vi "routes_n_m-optimised with LUT.vi"(6 "LUT in":T1[](array[typedef]), 8 "error in (no error)":errorcluster, 9 "recursivity counter in":u32, 10 "m = number of nodes (horizontal)":u64, 11 "n = number of nodes (vertical)":u64) -> (0 "error out":errorcluster, 1 "recursivity counter out":u32, 2 "no. of LUT elements":i32, 3 "r(n,m)= number of routes":u64, 4 "LUT out":T1[](array[typedef]))   [LabVIEW 2021, in "Project Euler.lvlib"]
uses:
  Project Euler.lvlib
  LUT_element.ctl
panel:
  # "Development\ncontrols/indicators useful for development and testing, but which are not outputs of the VI"
  # "Input\nInputs to the VI"
  # "Output\nOutputs of the VI"
  # "Description\n\nBlank VI with error handling case. \n\nSummarize the use of this VI in this space."
  # "r(15,15) = 40,116,600\nr(16,16) = 155,117,520\nr(17,17) = 601,080,390"
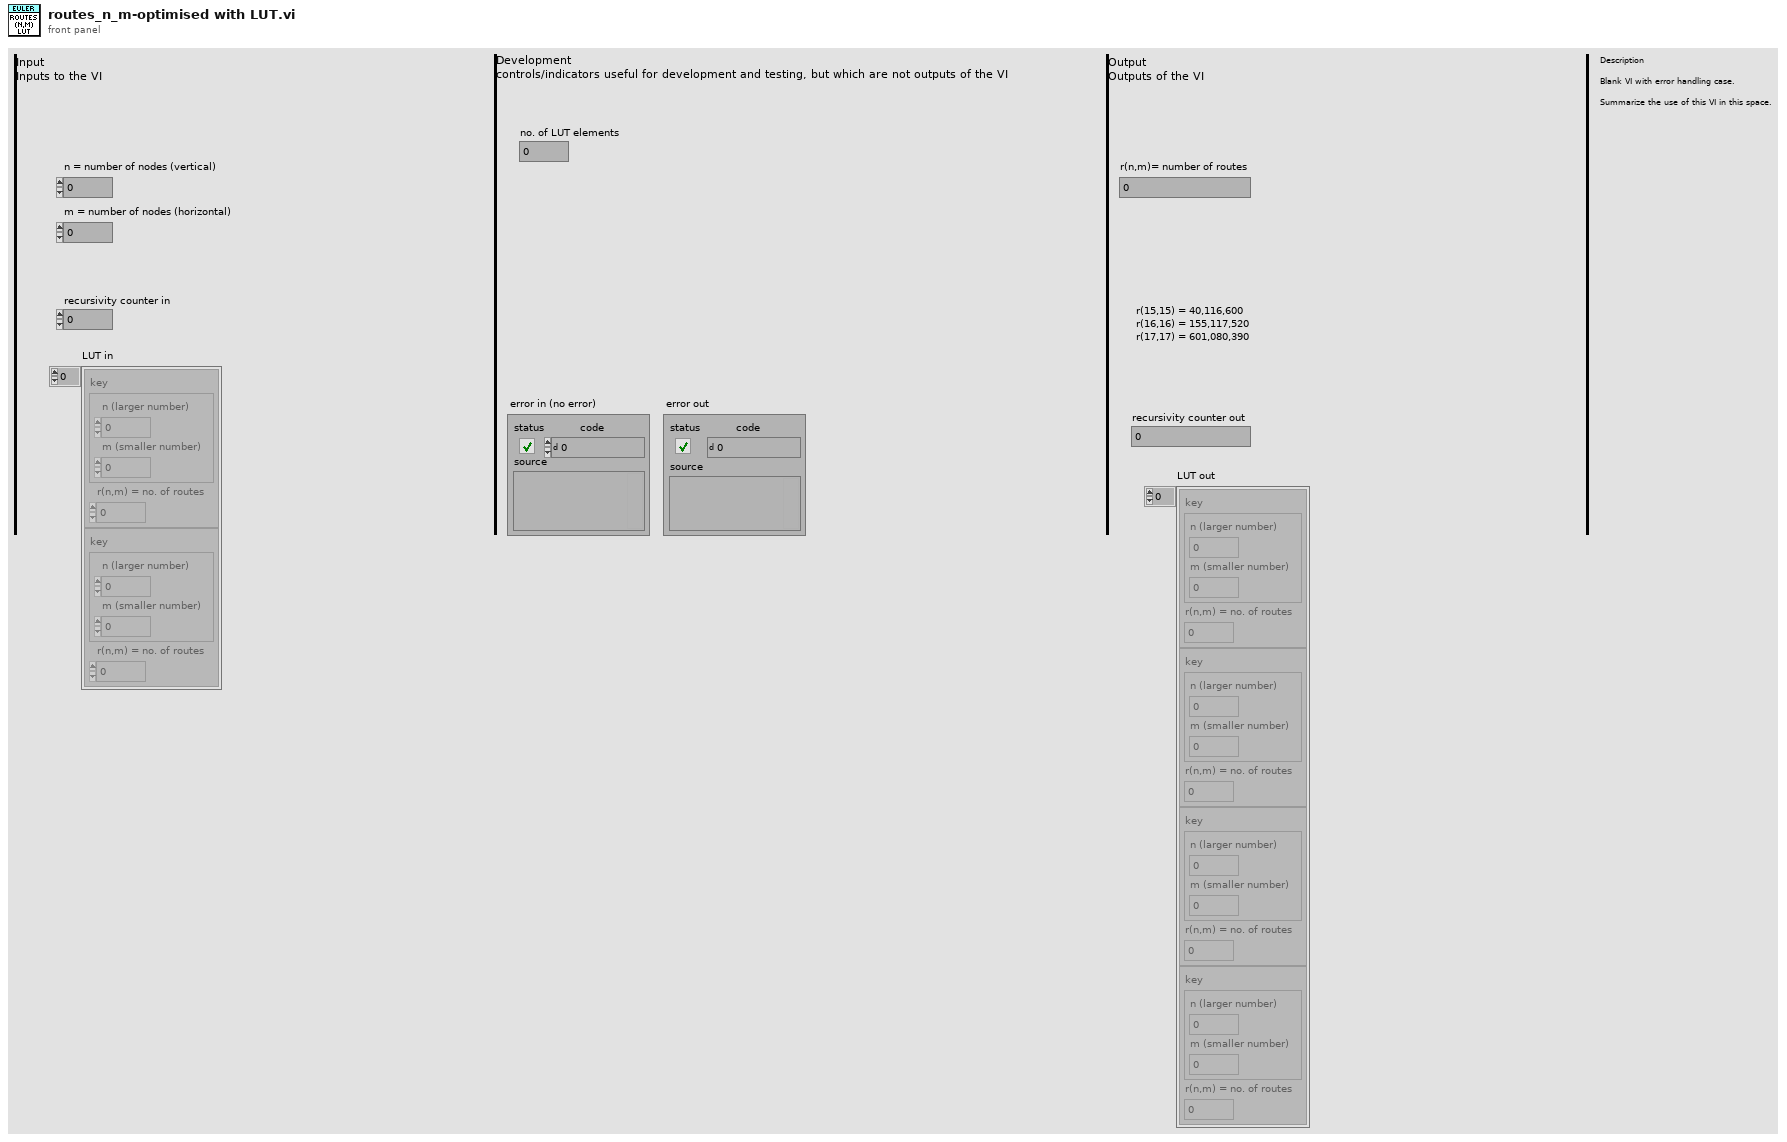
[diagram p1: front panel]
types:
  T1 = typedef "Project Euler.lvlib/LUT_element.ctl" = cluster{"key":cluster{"n (larger number)":u64, "m (smaller number)":u64}, "r(n,m) = no. of routes":u64}
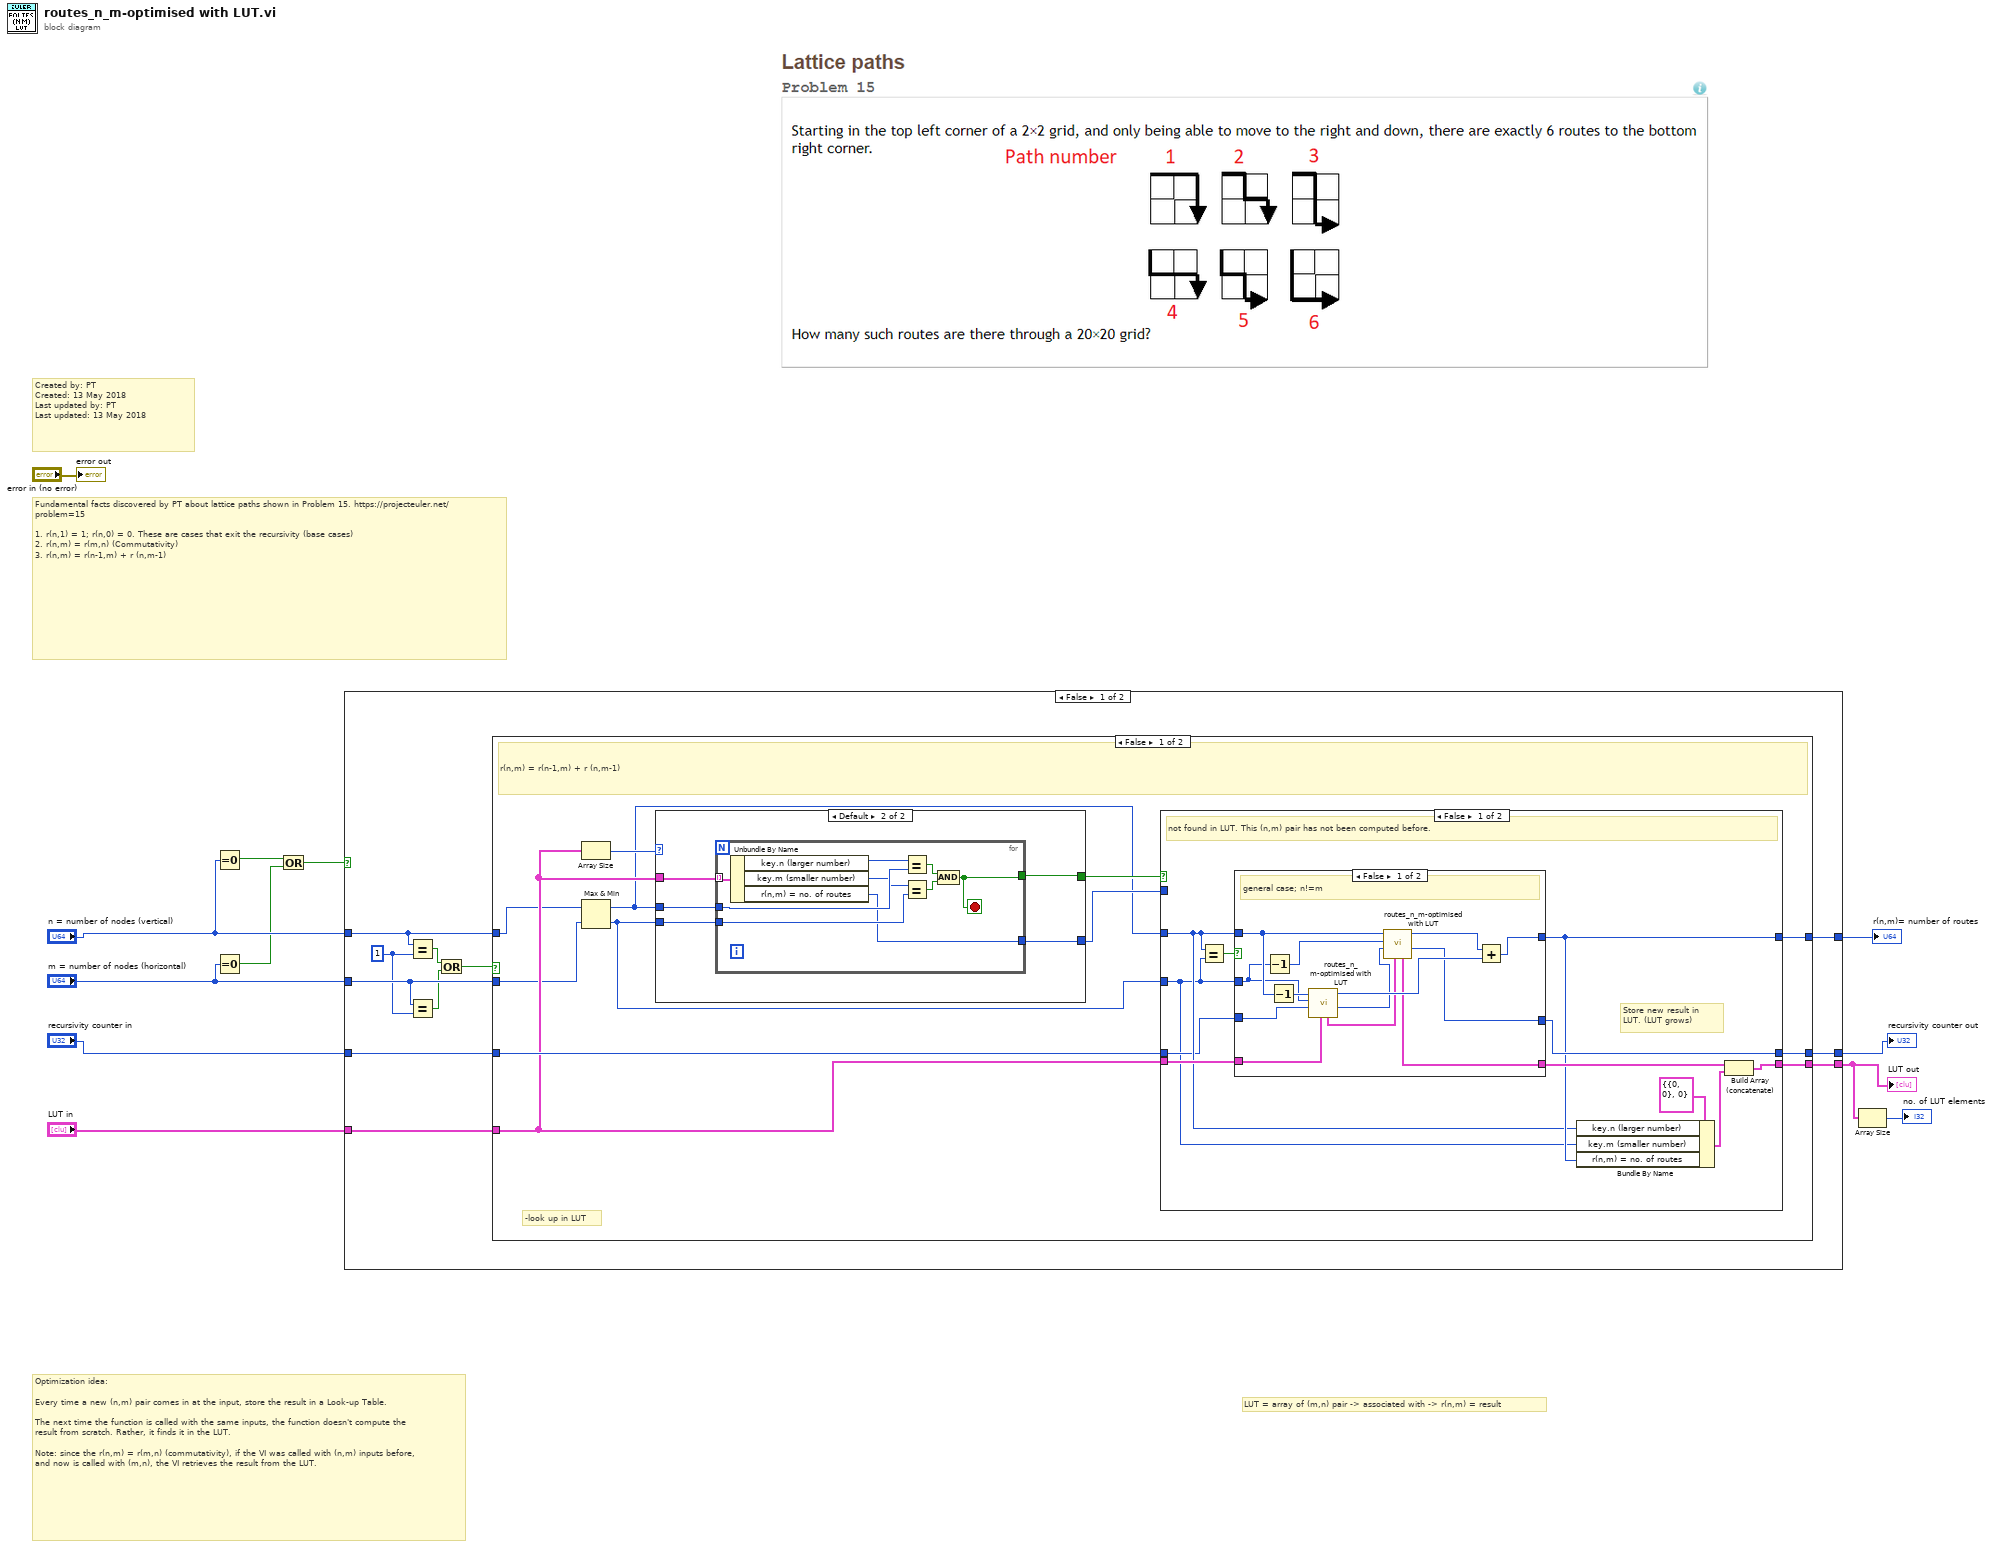
[diagram p0: block diagram]
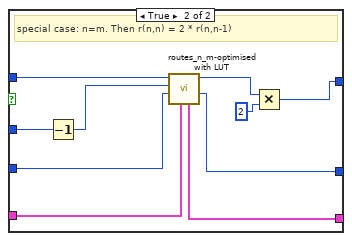
[diagram p3: hidden frame]
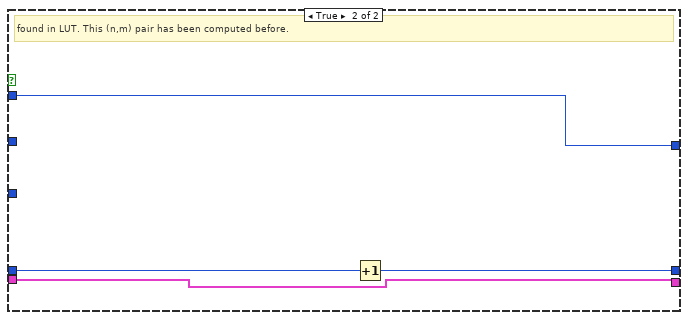
[diagram p4: hidden frame]
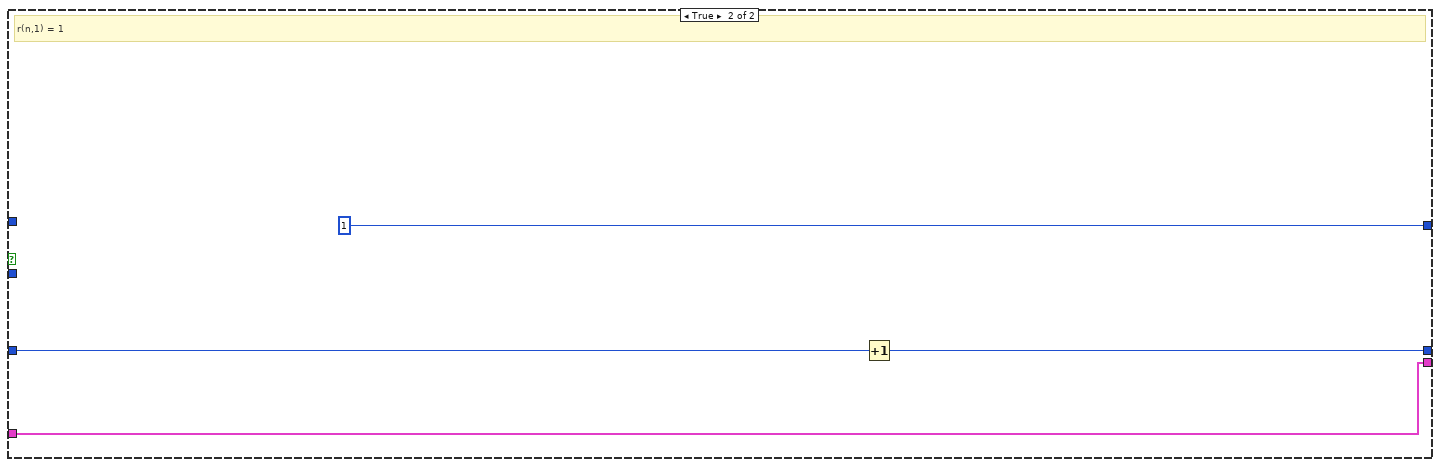
[diagram p5: hidden frame]
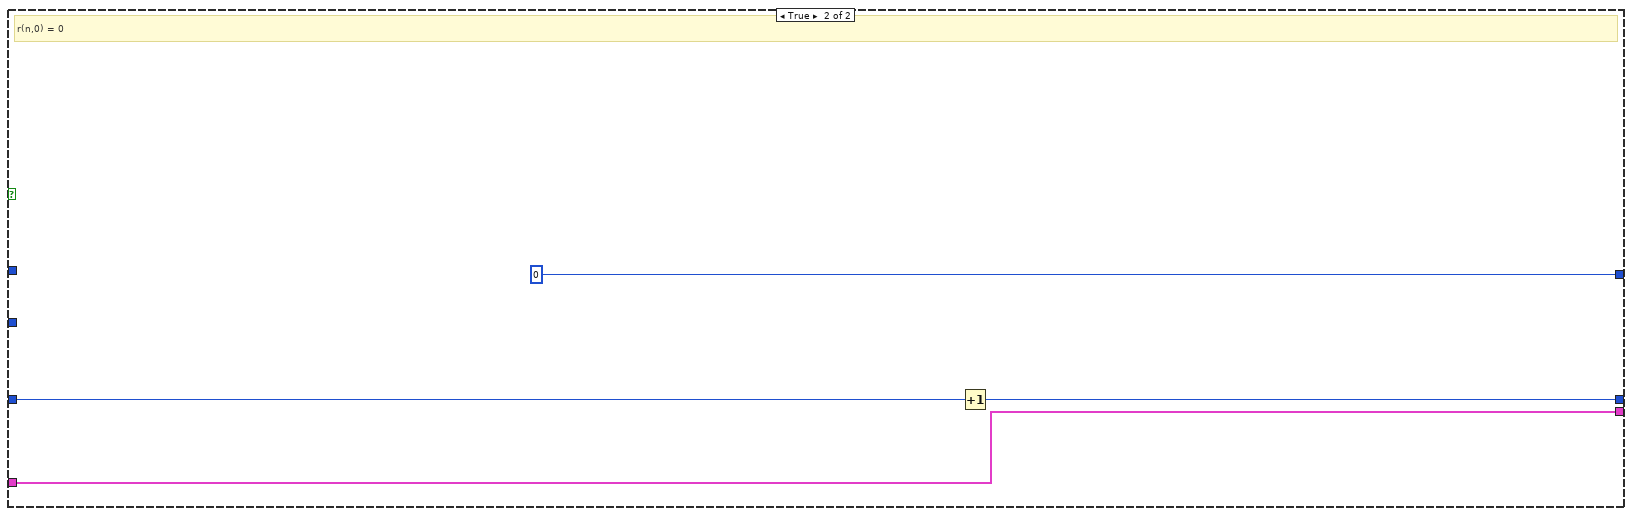
[diagram p6: hidden frame]
diagram:
  # "LUT = array of (m,n) pair -> associated with -> r(n,m) = result"
  # "Optimization idea:\n\nEvery time a new (n,m) pair comes in at the input, store the result in a Look-up Table.\n\nThe next time the function is called with the same inputs, the function doesn't compute the result from scratch. Rather, it finds it in the LUT.\n\nNote: since the r(n,m) = r(m,n) (commutativity), if the VI was called with (n,m) inputs before, and now is called with (m,n), the VI retrieves the result from the LUT."
  # "Fundamental facts discovered by PT about lattice paths shown in Problem 15. https://projecteuler.net/problem=15\n\n1. r(n,1) = 1; r(n,0) = 0. These are cases that exit the recursivity (base cases)\n2. r(n,m) = r(m,n) (Commutativity)\n3. r(n,m) = r(n-1,m) + r (n,m-1)"
  # "Created by: PT\nCreated: 13 May 2018\nLast updated by: PT\nLast updated: 13 May 2018"
  n1 = Equal To 0?(x="n = number of nodes (vertical)") -> (x = 0?=w8:bool)
  n2 = Equal To 0?(x="m = number of nodes (horizontal)") -> (x = 0?=w7:bool)
  n3 = Or(x=w8, y=w7) -> (x .or. y?=w6:bool)
  n4 = case shown="False" w6 {
    tunnel: [w23 u64 0 ("r(n,m)= number of routes")] -> w11
    tunnel: "n = number of nodes (vertical)" -> [w22 _]
    tunnel: "m = number of nodes (horizontal)" -> [w20 _]
    tunnel: "recursivity counter in" -> [w17 w94]
    tunnel: [w16 w93] -> w4
    tunnel: [w14 w92] -> w2
    tunnel: "LUT in" -> [w13 w92]
    frame False {
      w15 = u64 1 ("y")
      n5 = Equal?(x=w22, y=w15) -> (x = y?=w21:bool)
      n6 = Equal?(x=w20, y=w15) -> (x = y?=w19:bool)
      n7 = Or(x=w21, y=w19) -> (x .or. y?=w18:bool)
      n8 = case shown="False" w18 {
        tunnel: w22 -> [w27 _]
        tunnel: w20 -> [w25 _]
        tunnel: [w35 u64 1 ("r(n,m)= number of routes")] -> w23
        tunnel: w17 -> [w34 w90]
        tunnel: [w33 w89] -> w16
        tunnel: [w29 w88] -> w14
        tunnel: w13 -> [w28 w88]
        frame False {
          # "-look up in LUT"
          # "r(n,m) = r(n-1,m) + r (n,m-1)"
          n9 = Array Size(array=w28) -> (size(s)=w32:i32)
          n10 = Max & Min(x=w27, y=w25) -> (max(x,y)=w26:u64, min(x,y)=w24:u64)
          n11 = case shown="Default" w32 {
            tunnel: [_ w36] -> w31
            tunnel: w28 -> [_ w40]
            tunnel: w26 -> [_ w39]
            tunnel: w24 -> [_ w38]
            tunnel: [_ w37] -> w30
            frame 0 {
            }
            frame Default {
              n12 = for {
                tunnel: w40 -> [w49] mode=indexing
                tunnel: w39 -> [w47]
                tunnel: w38 -> [w45]
                tunnel: [w42] -> w37
                tunnel: [w41] -> w36
                stop <- w41 stop-if-true
                n13 = Unbundle By Name(w49) -> ("key.n (larger number)"=w48:u64, "key.m (smaller number)"=w46:u64, "r(n,m) = no. of routes"=w42:u64)
                n14 = Equal?(x=w48, y=w47) -> (x = y?=w44:bool)
                n15 = Equal?(x=w46, y=w45) -> (x = y?=w43:bool)
                n16 = And(x=w44, y=w43) -> (x .and. y?=w41:bool)
              }
            }
          }
          n17 = case shown="False" w31 {
            tunnel: [w53 w87] -> w35
            tunnel: w26 -> [w52 _]
            tunnel: w24 -> [w50 _]
            tunnel: w34 -> [w51 w85]
            tunnel: [w59 w86] -> w33
            tunnel: w30 -> [_ w87]
            tunnel: w28 -> [w58 w84]
            tunnel: [w56 w84] -> w29
            frame False {
              # "Store new result in LUT. (LUT grows)"
              # "not found in LUT. This (n,m) pair has not been computed before."
              n18 = Equal?(x=w52, y=w50) -> (x = y?=w60:bool)
              n19 = case shown="False" w60 {
                tunnel: w52 -> [w70 w83]
                tunnel: w50 -> [w68 w82]
                tunnel: [w67 w78] -> w53
                tunnel: w51 -> [w66 w77]
                tunnel: [w64 w76] -> w59
                tunnel: w58 -> [w63 w75]
                tunnel: [w61 w74] -> w57
                frame False {
                  # "general case; n!=m"
                  n20 = Decrement(x=w68) -> (x-1=w73:u64)
                  n21 = Decrement(x=w70) -> (x-1=w69:u64)
                  n22 = call "routes_n_m-optimised with LUT.vi"("LUT in"=w63, "recursivity counter in"=w66, "m = number of nodes (horizontal)"=w68, "n = number of nodes (vertical)"=w69) -> ("recursivity counter out"=w65:u32, "r(n,m)= number of routes"=w71:u64, "LUT out"=w62:T1[])  [unwired: 3 in, 2 out]
                  n23 = call "routes_n_m-optimised with LUT.vi"("LUT in"=w62, "recursivity counter in"=w65, "m = number of nodes (horizontal)"=w73, "n = number of nodes (vertical)"=w70) -> ("recursivity counter out"=w64:u32, "r(n,m)= number of routes"=w72:u64, "LUT out"=w61:T1[])  [unwired: 3 in, 2 out]
                  n24 = Add(x=w72, y=w71) -> (x+y=w67:u64)
                }
                frame True {
                  # "special case: n=m. Then r(n,n) = 2 * r(n,n-1)"
                  n25 = Decrement(x=w82) -> (x-1=w81:u64)
                  n26 = call "routes_n_m-optimised with LUT.vi"("LUT in"=w75, "recursivity counter in"=w77, "m = number of nodes (horizontal)"=w81, "n = number of nodes (vertical)"=w83) -> ("recursivity counter out"=w76:u32, "r(n,m)= number of routes"=w80:u64, "LUT out"=w74:T1[])  [unwired: 3 in, 2 out]
                  n27 = Multiply(x=w80, y=u64 2) -> (x*y=w78:u64)
                }
              }
              n28 = Bundle By Name(cluster=T1 {"key"={"n (larger number)"=0, "m (smaller number)"=0}, "r(n,m) = no. of routes"=0} ("LUT_element"), "key.n (larger number)"=w52, "key.m (smaller number)"=w50, "r(n,m) = no. of routes"=w53) -> (w54:T1)
              n29 = Build Array (concatenate)(w57, w54) -> (w56:T1[])
            }
            frame True {
              # "found in LUT. This (n,m) pair has been computed before."
              n30 = Increment(x=w85) -> (x+1=w86:u32)
            }
          }
        }
        frame True {
          # "r(n,1) = 1"
          n31 = Increment(x=w90) -> (x+1=w89:u32)
        }
      }
    }
    frame True {
      # "r(n,0) = 0"
      n32 = Increment(x=w94) -> (x+1=w93:u32)
    }
  }
  "r(n,m)= number of routes" <- w11
  "recursivity counter out" <- w4
  "LUT out" <- w2
  n33 = Array Size(array=w2) -> (size(s)=→"no. of LUT elements":i32)
  "error out" <- "error in (no error)"
